vi "Measure Voltage.vi"(8 "error in (no error)":errorcluster, 11 "DAQ in":refnum<class "DAQ.lvclass">) -> (0 "error out":errorcluster, 2 "Voltage (V)":dbl, 3 "DAQ out":refnum<class "DAQ.lvclass">)   [LabVIEW 2024, in "HAL_Example.lvlib" / "DAQ.lvclass"]
uses:
  DAQ.lvclass
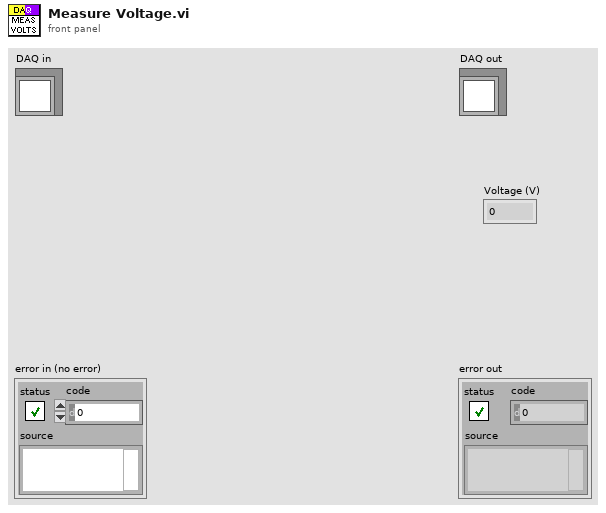
[diagram p1: front panel]
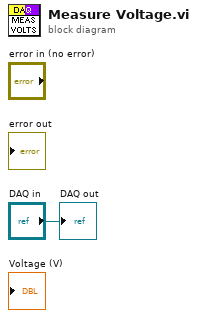
[diagram p0: block diagram]
diagram:
  "DAQ out" <- "DAQ in"
